vi "test - List SysLevel CSM Modules.vi"(8 "error in (no error)":errorcluster, 11 "TestCase in":refnum<class "testcase-Basic-Function.lvclass">) -> (0 "error out":errorcluster, 3 "TestCase out":refnum<class "testcase-Basic-Function.lvclass">)   [LabVIEW 2017, in "testcase-Basic-Function.lvclass"]
uses:
  testcase-Basic-Function.lvclass
  testcase-Basic-Function.lvclass/testcase-Basic-Function.ctl
  src/user.lib/_NEVSTOP/Communicable State Machine(CSM)/_Support/Error/CSM Invalid Name Error.vi
  <vilib>/addons/_JKI Toolkits/VI Tester/TestCase.llb/TestCase.lvclass
  src/user.lib/_NEVSTOP/Communicable State Machine(CSM)/Communicable State Machine.lvlib
  C:/Program Files (x86)/National Instruments/LabVIEW 2017/vi.lib/addons/_JKI Toolkits/VI Tester/TestCase.llb/TestCase.lvclass
panel:
  out "error out 2":errorcluster
  out "CSM Name(marked as Sysetem-Level Module)":string
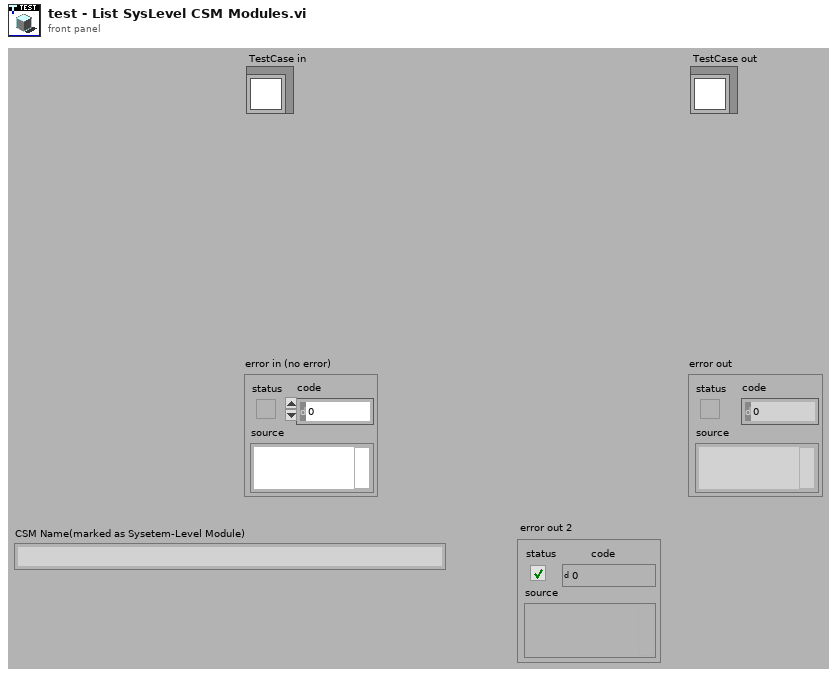
[diagram p1: front panel]
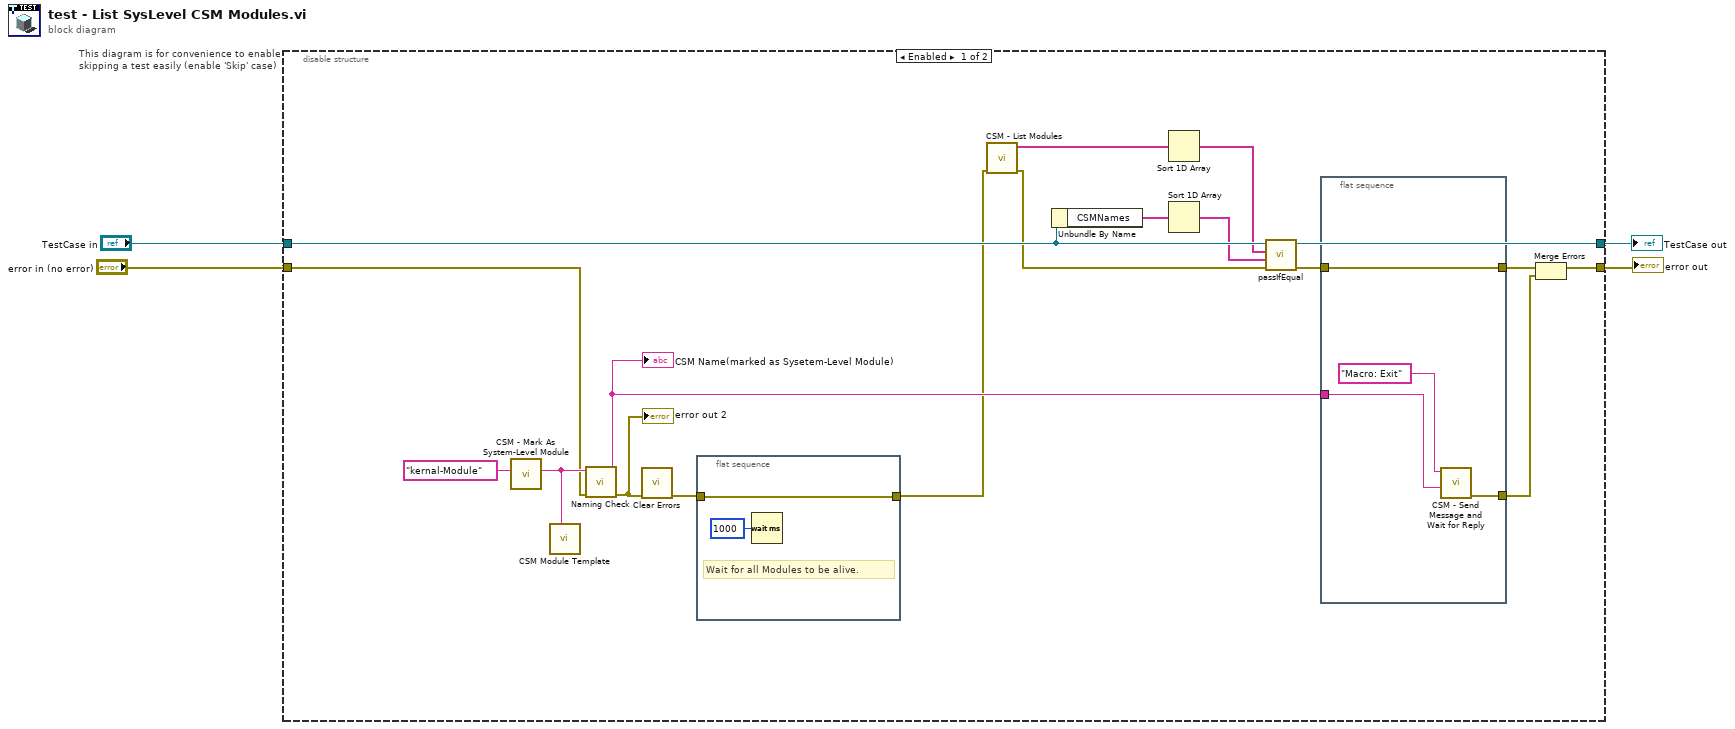
[diagram p0: block diagram]
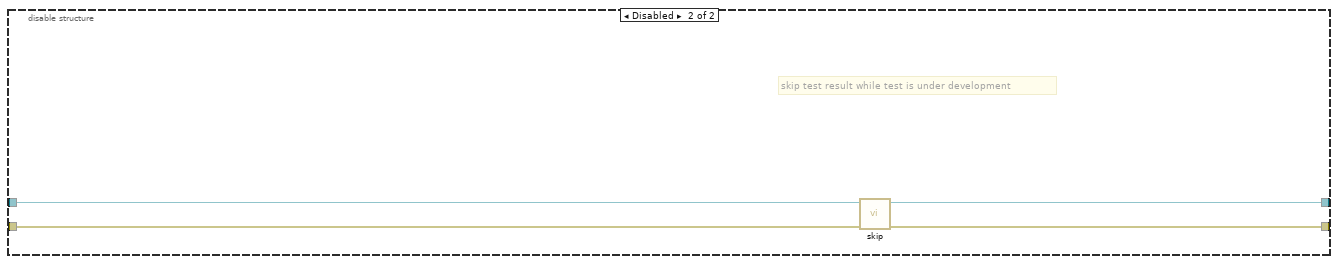
[diagram p2: hidden frame]
diagram:
  n1 = disable-structure "This diagram is for convenience to enable skipping a test easily (enable 'Skip' case)" shown="Enabled" {
    disable-tunnel: "TestCase in" -> [w20 w32]
    disable-tunnel: [w22 w30] -> w1
    disable-tunnel: [w8 w31] -> w3
    disable-tunnel: "error in (no error)" -> [w10 w29]
    frame Enabled {
      n2 = call "CSM - Mark As System-Level Module.vi"("CSM Name"="kernal-Module") -> ("CSM Name (Marked As Sysetem-Level Module)"=w14:string)  [unwired: 9 in]
      n3 = call "CSM Module Template.vi"("Name (\"\" to Use UUID)"=w14) -> ()  [unwired: 11 in]
      n4 = call "Naming Check.vi"("error in (no error)"=w10, "Name (\"\" to Use UUID)"=w14) -> ("error out"=w13:errorcluster, "Name (Dup)"=w11:string)  [unwired: 8 in]
      "CSM Name(marked as Sysetem-Level Module)" <- w11
      "error out 2" <- w13
      n5 = call <vilib>:"Clear Errors.vi"("error in (no error)"=w13) -> ("error out"=w12:errorcluster)  [unwired: 5 in, 1 out]
      n6 = flat-sequence {
        tunnel: [w27] -> w9
        tunnel: w12 -> [w27]
        frame #0 {
          # "Wait for all Modules to be alive."
          n7 = Wait (ms)(milliseconds to wait=u32 1000) -> ()  [unwired: 1 out]
        }
      }
      n8 = call "CSM - List Modules.vi"("Error In"=w9) -> ("error out"=w19:errorcluster, "Module Names"=w21:string[])  [unwired: 9 in]
      n9 = Unbundle By Name(w20) -> ("CSMNames"=w18:string[])
      n10 = Sort 1D Array(array=w21) -> (sorted array=w17:string[])
      n11 = Sort 1D Array(array=w18) -> (sorted array=w16:string[])
      n12 = call-dynamic "passIfEqual.vi"("error in (no error)"=w19, "y"=w16, "x"=w17, "TestCase in"=w20) -> ("error out"=w5:errorcluster, "TestCase out"=w22:refnum<class "testcase-Basic-Function.lvclass">)  [unwired: 6 in]
      n13 = flat-sequence {
        tunnel: w11 -> [w26]
        tunnel: [w24] -> w7
        tunnel: [w23] -> w6
        tunnel: w5 -> [w23]
        frame #0 {
          n14 = call "CSM - Send Message and Wait for Reply.vi"("Target Module"=w26, "State"="Macro: Exit" ("CSM Name")) -> ("error out"=w24:errorcluster)  [unwired: 7 in, 2 out]
        }
      }
      n15 = Merge Errors(w6, w7) -> (w8:errorcluster)
    }
    frame Disabled {
      # "skip test result while test is under development"
      n16 = call <vilib>:"skip.vi"("error in (no error)"=w29, "TestCase in"=w32) -> ("error out"=w31:errorcluster, "TestCase out"=w30:refnum<class "testcase-Basic-Function.lvclass">)  [unwired: 8 in]
    }
  }
  "error out" <- w3
  "TestCase out" <- w1
